vi "BasicControlPathAndType_Tests.vi"(11 "error in (no error)":errorcluster) -> (15 "error out":errorcluster)   [LabVIEW 2016, in "DronaTest.lvlib"]
uses:
  DronaTest.lvlib
  APIs/Stimulus/ControlValue/ValueSignalByPathString.vi
  APIs/Assert/AssertControlValue/Equal.vi
  <vilib>/addons/_JKI Toolkits/Caraya/classes/Test/Test.lvclass
  Drona.lvlib
  APIs/Assert/AssertControlValue/AssertControlValue.lvlib
  APIs/Stimulus/ControlValue/ControlValue.lvlib
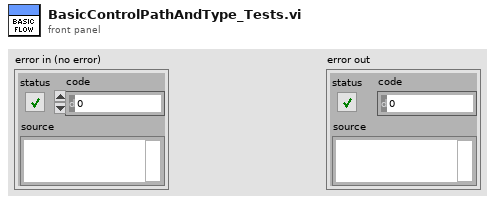
[diagram p1: front panel]
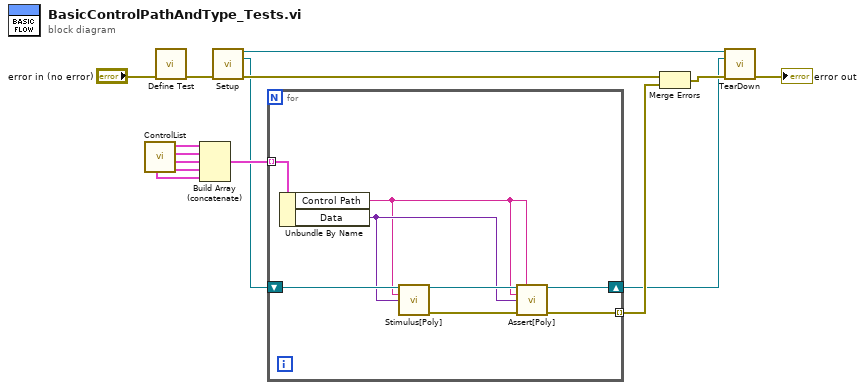
[diagram p0: block diagram]
diagram:
  n1 = call "ControlList.vi"() -> ("Tab Control"=w7:cluster{"Control Path":string, "Data":variant}[], "BigCluster"=w8:cluster{"Control Path":string, "Data":variant}[], "Cluster"=w9:cluster{"Control Path":string, "Data":variant}[], "Basic"=w12:cluster{"Control Path":string, "Data":variant}[], "BasicArray"=w6:cluster{"Control Path":string, "Data":variant}[])  [unwired: 6 in, 1 out]
  n2 = call <vilib>:"Define Test.vi"("error in (no error)"="error in (no error)") -> ("error out"=w11:errorcluster)  [unwired: 10 in]
  n3 = Build Array (concatenate)(w12, w9, w8, w7, w6) -> (w10:cluster{"Control Path":string, "Data":variant}[])
  n4 = call "Setup.vi"("error in (no error)"=w11) -> ("Application Ref"=w1:refnum<vi>, "VI out"=w2:refnum<vi>, "error out"=w5:errorcluster)  [unwired: 12 in]
  n5 = for {
    shift-right: [w23] -> w3
    shift-left: w2 -> [w19]
    tunnel: [w16] -> w15 mode=indexing
    tunnel: w10 -> [w20] mode=indexing
    n6 = Unbundle By Name(w20) -> ("Control Path"=w17:string, "Data"=w18:variant)
    n7 = call-poly "Stimulus[Poly].vi"("VI Reference In"=w19, "Control Path"=w17, "Value (Signaling)"=w18) -> ("VI Reference Out"=w21:refnum<vi>, "error out"=w22:errorcluster)  [unwired: 11 in]
    n8 = call-poly "Assert[Poly].vi"("VI Reference In"=w21, "Test Label"=w17, "Control Path"=w17, "Control Value"=w18, "Error In"=w22) -> ("VI Reference Out"=w23:refnum<vi>, "Error Out"=w16:errorcluster)  [unwired: 9 in]
  }
  n9 = Merge Errors(w5, w15) -> (w13:errorcluster)
  n10 = call "TearDown.vi"("Application Ref"=w1, "VI in"=w3, "error in (no error)"=w13) -> ("error out"=→"error out":errorcluster)  [unwired: 12 in]
